vi "Error Processor.vi"(8 "error in (no error)":errorcluster, 11 "Template Internal uService in":refnum<class "Run Config Manager.lvclass">) -> (0 "error out":errorcluster, 3 "Template Internal uService out":refnum<class "Run Config Manager.lvclass">)   [LabVIEW 2026, in "TALOS.lvlib" / "Run Config Manager.lvlib" / "Run Config Manager.lvclass"]
doc: "Use this VI to process all the error that are solvable inside this specific uService. Whatever is not possible to process, let it leave this VI and it will be processed by the Error Manager of the Distributed System."
uses:
  Run Config Manager.lvclass
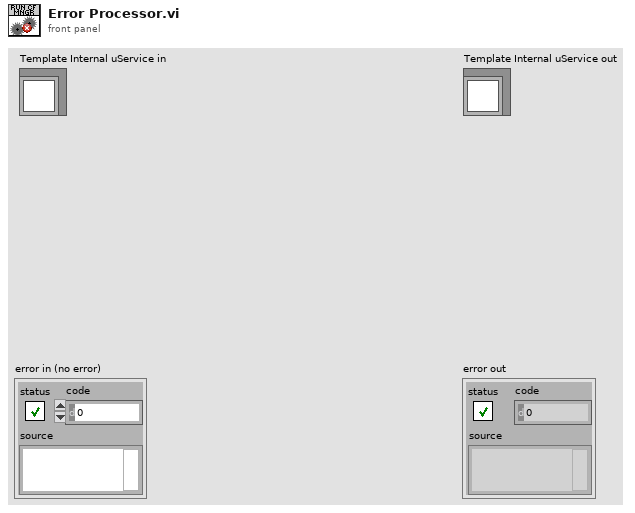
[diagram p1: front panel]
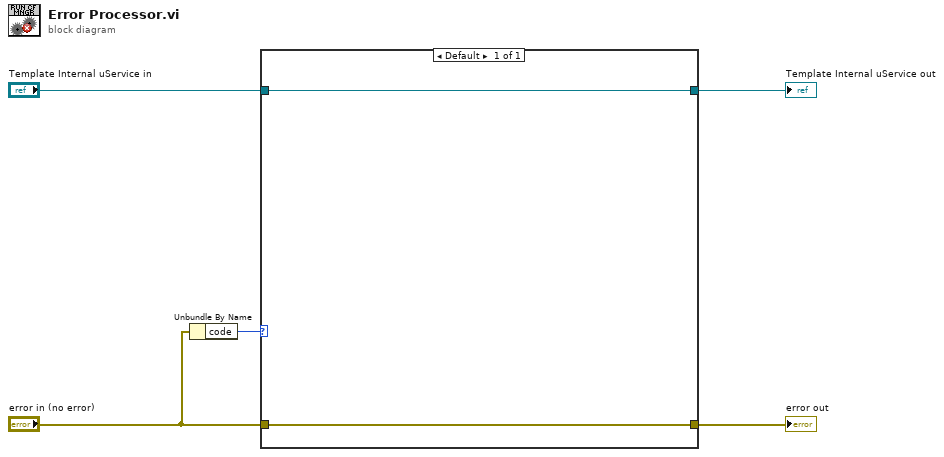
[diagram p0: block diagram]
diagram:
  n1 = Unbundle By Name("error in (no error)") -> ("code"=w1:i32)
  n2 = case shown="Default" w1 {
    tunnel: "error in (no error)" -> [w7]
    tunnel: [w7] -> w3
    tunnel: "Template Internal uService in" -> [w6]
    tunnel: [w6] -> w2
    frame Default {
    }
  }
  "error out" <- w3
  "Template Internal uService out" <- w2
